vi "build xml file path (AIM).vi"(8 "additional string(\"\")":string, 10 "Filetype":enum16{"Hardware", "Parameter"}(ring), 11 "Database Filepath in":path) -> (3 "xml path out":path)   [LabVIEW 2020]
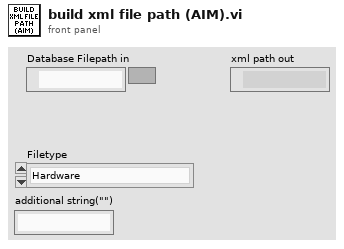
[diagram p1: front panel]
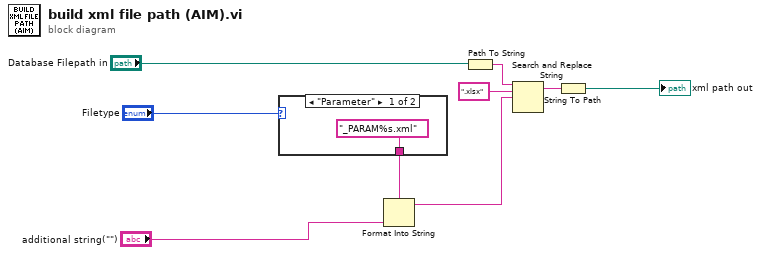
[diagram p0: block diagram]
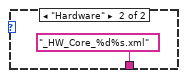
[diagram p2: hidden frame]
diagram:
  n1 = case shown="\"Parameter\"" "Filetype" {
    tunnel: ["_PARAM%s.xml" ("format string") "_HW_Core_%d%s.xml" ("format string")] -> w7
    frame "Parameter" {
    }
    frame "Hardware" {
    }
  }
  n2 = Format Into String(format string=w7, "additional string(\"\")") -> (resulting string=w4:string)  [unwired: 2 in, 1 out]
  n3 = Path To String(path="Database Filepath in") -> (string=w2:string)
  n4 = Search and Replace String(input string=w2, search string=".xlsx", replace string=w4) -> (result string=w8:string)  [unwired: 5 in, 3 out]
  n5 = String To Path(string=w8) -> (path=→"xml path out":path)
